vi "Do.vi"(8 "error in (no error)":cluster{"状态":bool, "代码":i32, "源":string} caption="错误输入（无错误）", 10 "操作者输入":refnum<class "Actor.lvclass">, 11 "记录事件消息":refnum<class "Log Event Msg.lvclass">) -> (0 "error out":cluster{"状态":bool, "代码":i32, "源":string} caption="错误输出", 2 "操作者输出":refnum<class "Actor.lvclass">)   [LabVIEW 2013, in "操作者框架.lvlib" / "Log Event Msg.lvclass"]
uses:
  Log Event Msg.lvclass
  <vilib>/ActorFramework/Actor/Actor.lvclass
  Log Event Msg.lvclass/Log Event Msg.ctl
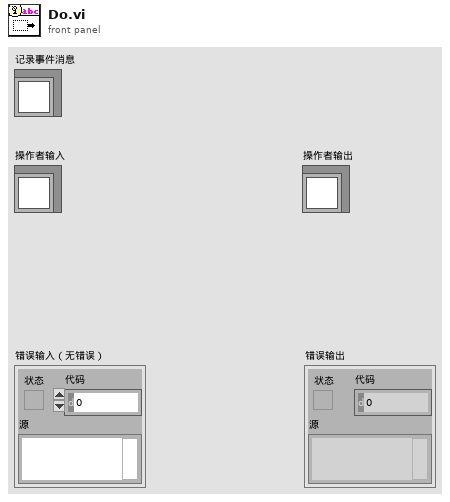
[diagram p1: front panel]
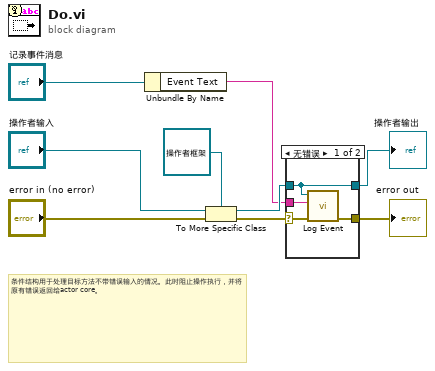
[diagram p0: block diagram]
diagram:
  # "条件结构用于处理目标方法不带错误输入的情况。此时阻止操作执行，并将原有错误返回给actor core。"
  n1 = Unbundle By Name("记录事件消息") -> ("Event Text"=w2:string)
  n2 = To More Specific Class(target class=refnum<class "操作者框架.lvclass"> refnum ("Actor in"), reference="操作者输入", error in="error in (no error)") -> (specific class reference=w9:refnum<class "操作者框架.lvclass">, error out=w5:errorcluster)
  n3 = case shown="无错误" w5 {
    selector: w5 -> [w12 w15]
    tunnel: w9 -> [w10 w14]
    tunnel: [w13 w15] -> w4
    tunnel: [w10 w14] -> w3
    tunnel: w2 -> [w11 _]
    frame No Error {
      n4 = call "Log Event.vi"("error in (no error)"=w12, "事件文本"=w11, "操作者框架输入"=w10) -> ("error out"=w13:cluster{"状态":bool, "代码":i32, "源":string})  [unwired: 8 in]
    }
    frame Error {
    }
  }
  "error out" <- w4
  "操作者输出" <- w3
